vi "WinOption.vi"(8 "error in":errorcluster) -> (0 "error out":errorcluster)   [LabVIEW 2016]
uses:
  Ctl/Option.ctl
panel:
  in  "管理员登录":bool
  in  "选项卡控件":enum32{"基本配置", "流程配置"}(tab)
  in  "Caldata":T1={"分辨率"="", "Fps"=0, "工单号"="", "操作人"="", "增益模式"=enum."高低增益切换", "黑体设定温度1"=0.0, "温差范围1"=0.0, "出图到测温等待时间"=0.0, "调焦数值min"=0, "盲元阈值"=0.0, "盲元采样帧数"=0, "调焦数值min2"=0, "黑体设定温度2"=0.0, "温差范围2"=0.0, "ID选择"=enum."新ID", "快门时间间隔设置"={"快门第一次延时时间"=200, "快门第二次延时时间"=200, "切换增益后快门第一次延时时间"=200, "切换增益后快门第二次延时时间"=200}, "产品名"="Tiny1_C", "镜头"="02011X", "测温功能"="WR", "产品料号"="", "打印机VISA"="", "焦距选择"=enum."Radio Selection 1", "工位"="0001", "服务器保存地址"=path ""}
  in  "Exit":bool
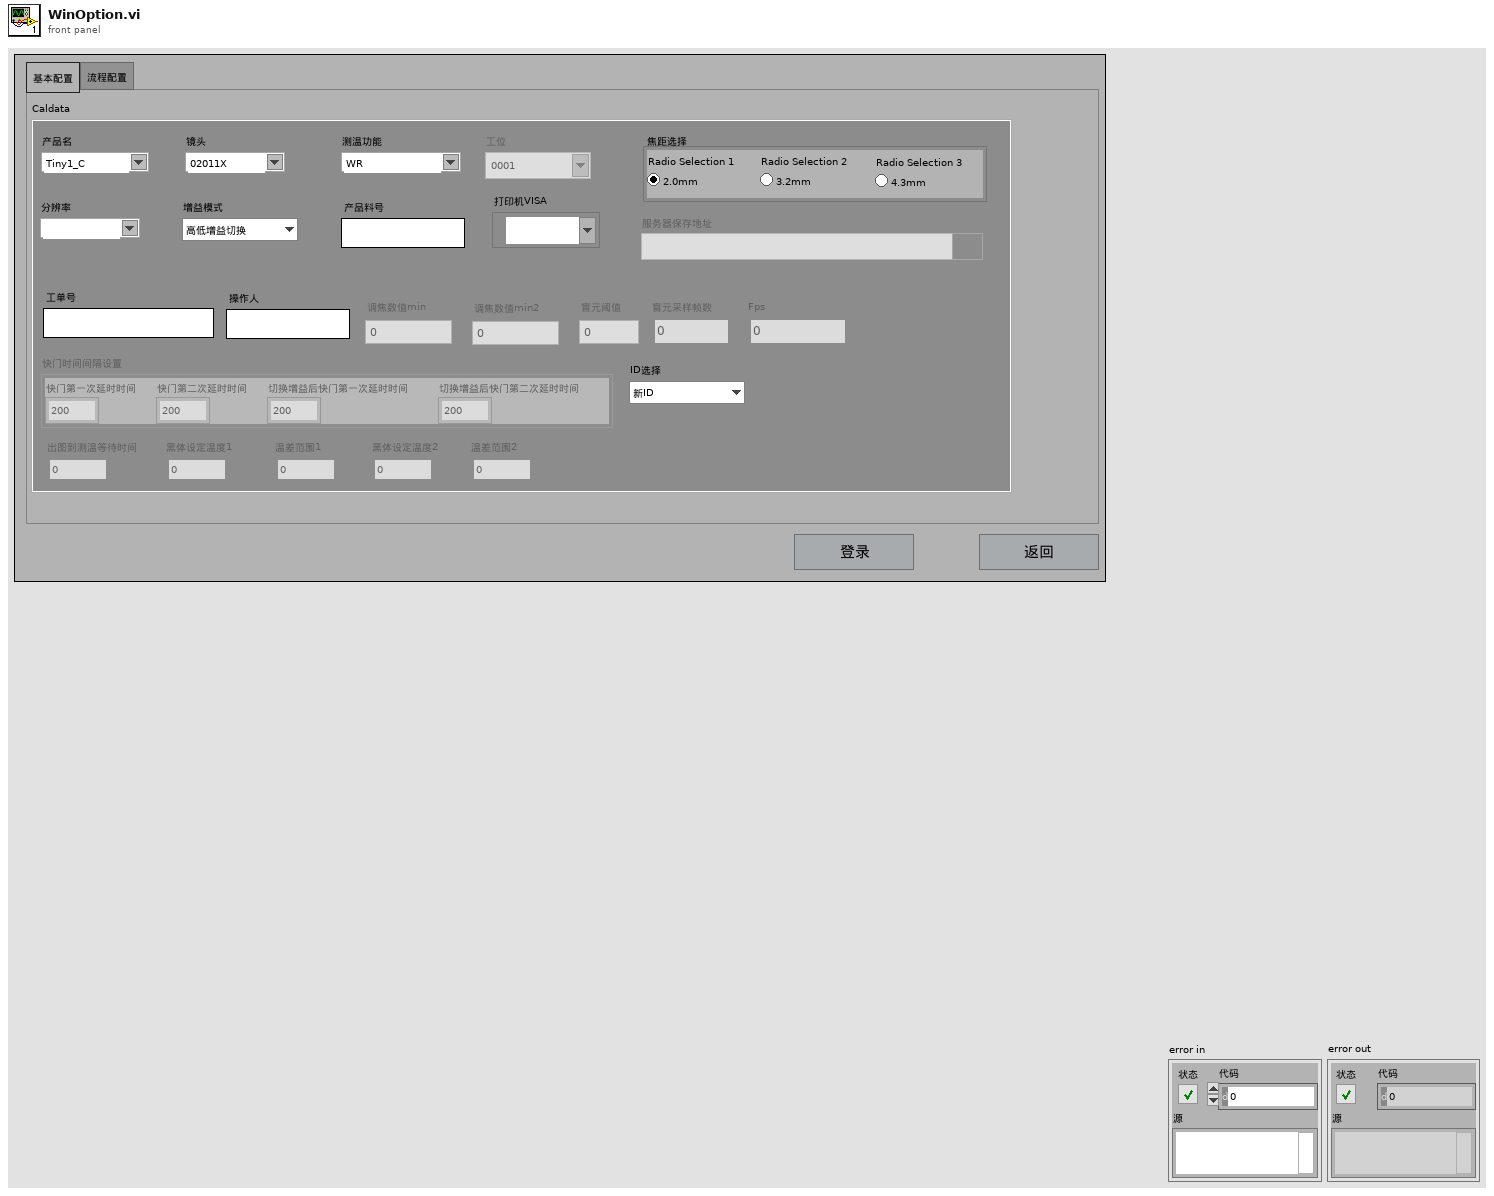
[diagram p1: front panel]
types:
  T1 = typedef "Option.ctl" = cluster{"分辨率":string, "Fps":u16, "工单号":string, "操作人":string, "增益模式":enum16{"高低增益切换", "高增益"}, "黑体设定温度1":dbl, "温差范围1":dbl, "出图到测温等待时间":dbl, "调焦数值min":i32, "盲元阈值":dbl, "盲元采样帧数":u16, "调焦数值min2":i32, "黑体设定温度2":dbl, "温差范围2":dbl, "ID选择":enum16{"旧ID", "新ID"}, "快门时间间隔设置":cluster{"快门第一次延时时间":u16, "快门第二次延时时间":u16, "切换增益后快门第一次延时时间":u16, "切换增益后快门第二次延时时间":u16}, "产品名":string, "镜头":string, "测温功能":string, "产品料号":string, "打印机VISA":refnum<visa-resource-name>, "焦距选择":enum32{"Radio Selection 1", "Radio Selection 2", "Radio Selection 3"}, "工位":string, "服务器保存地址":path}
  T2 = cluster{"CalData":path, "Datasave":path, "Data":path}
  T3 = enum8{"Enabled", "Disabled", "Disabled and Grayed Out"}
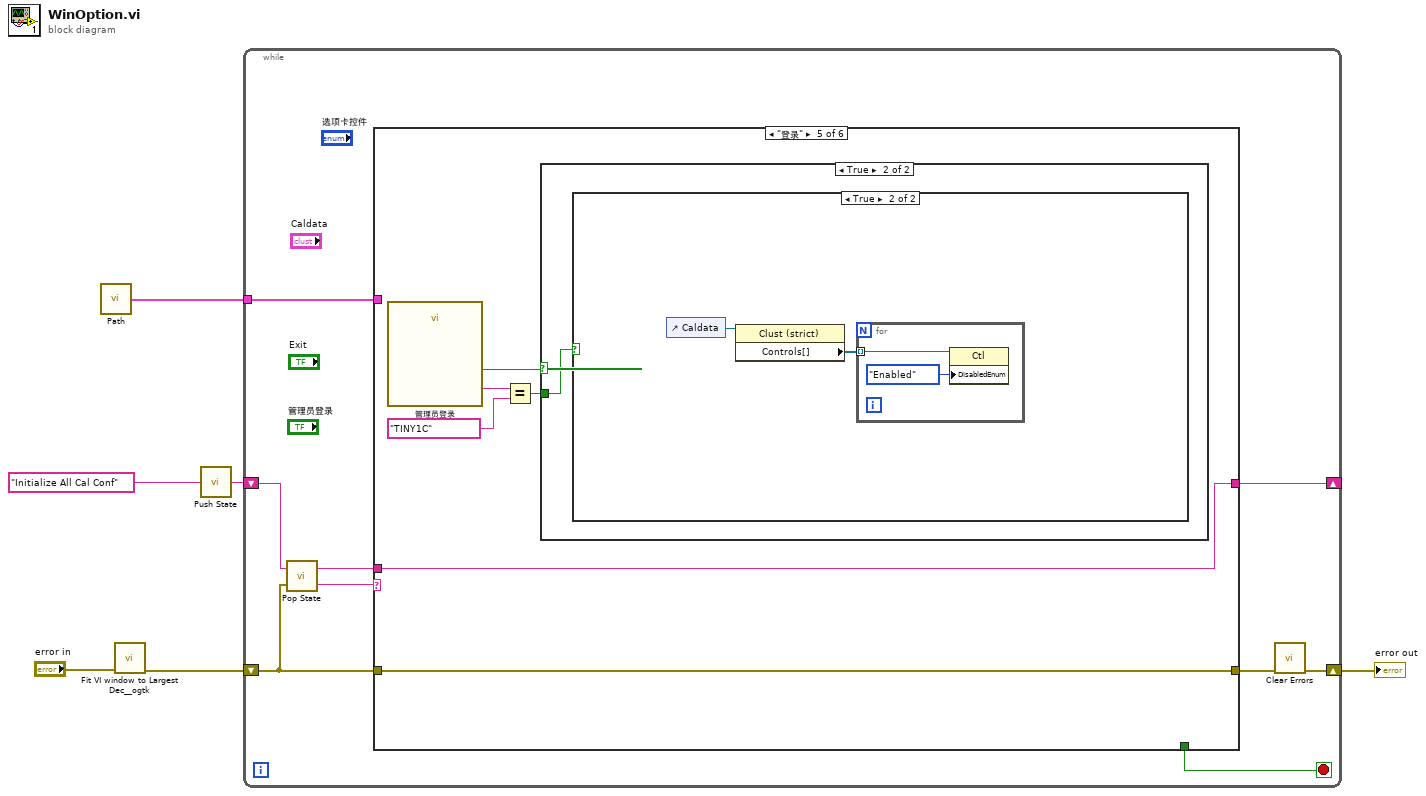
[diagram p0: block diagram]
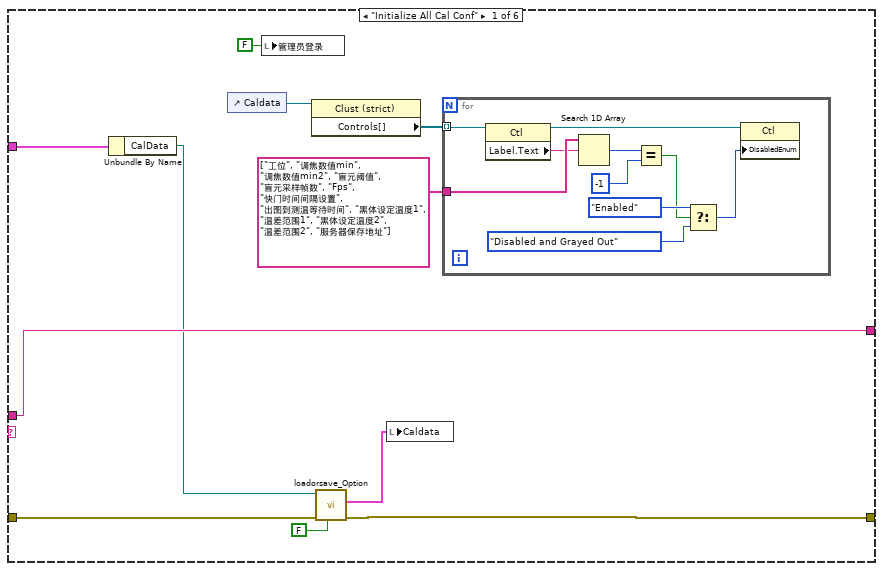
[diagram p2: hidden frame]
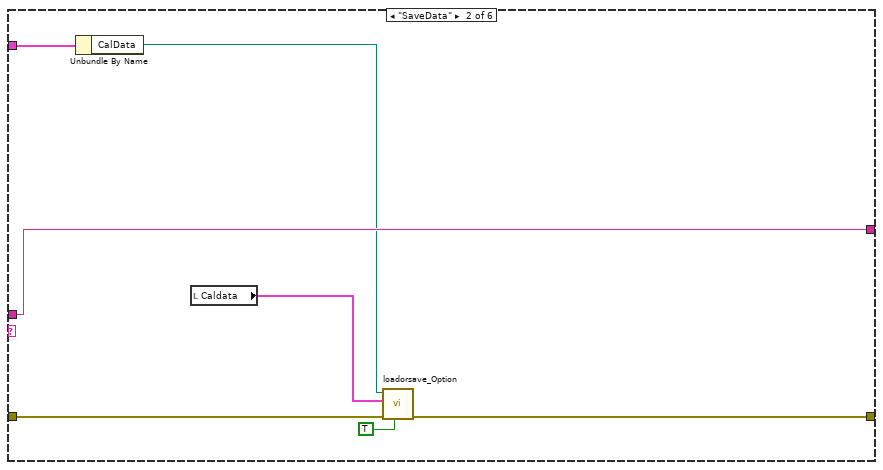
[diagram p3: hidden frame]
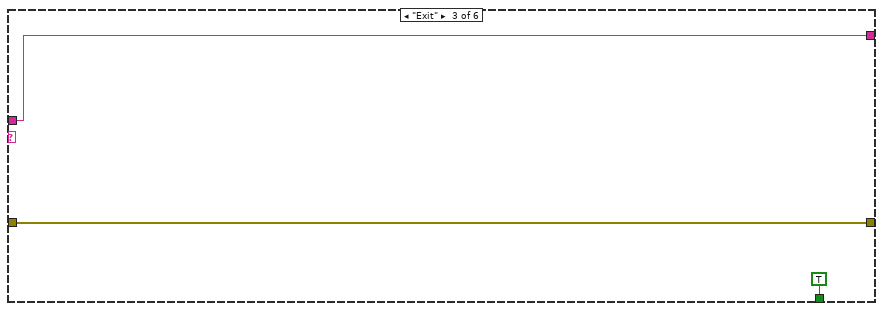
[diagram p4: hidden frame]
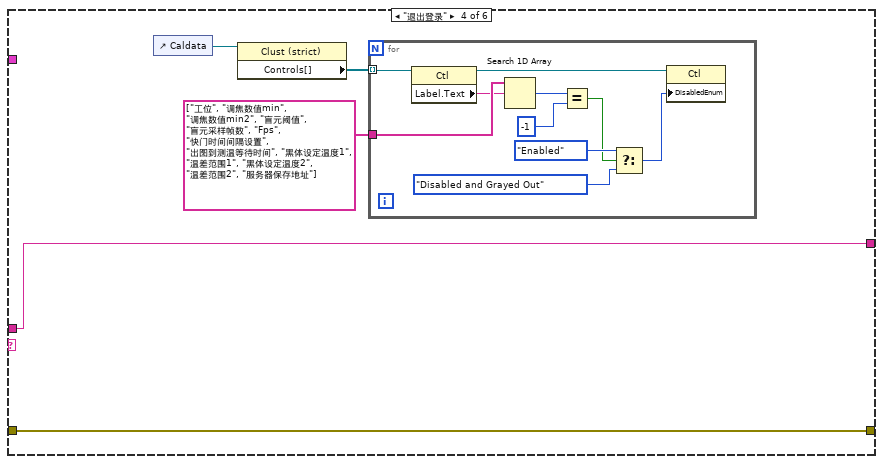
[diagram p5: hidden frame]
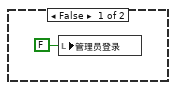
[diagram p6: hidden frame]
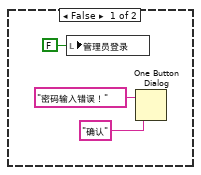
[diagram p7: hidden frame]
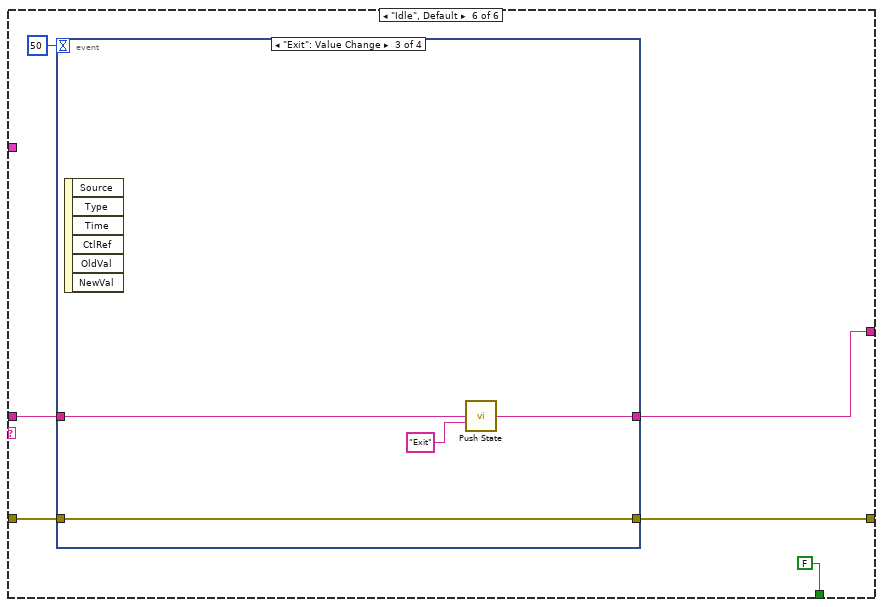
[diagram p8: hidden frame]
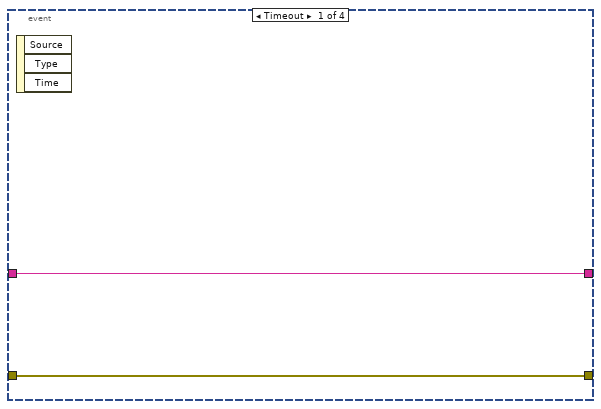
[diagram p9: hidden frame]
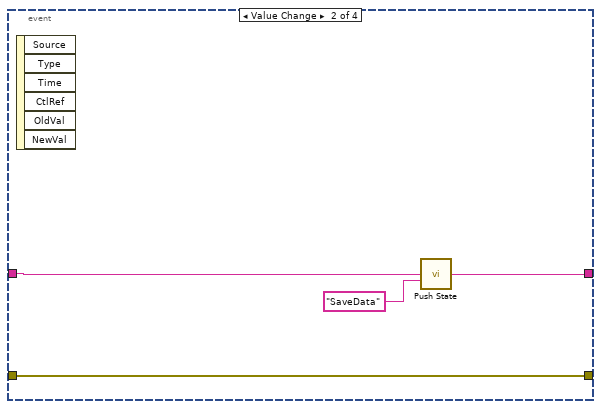
[diagram p10: hidden frame]
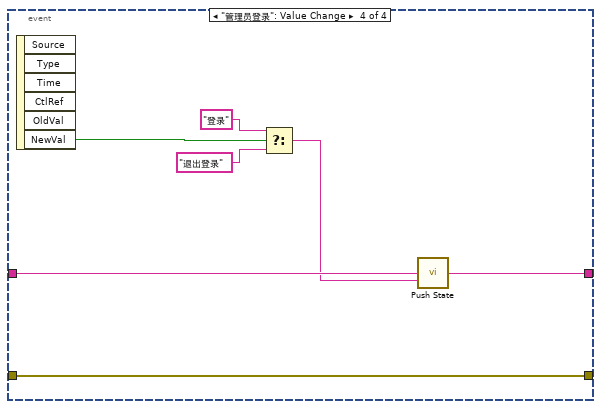
[diagram p11: hidden frame]
diagram:
  n1 = call "Path.vi"() -> ("path"=w1:T2)  [unwired: 9 in]
  n2 = call "Fit VI window to Largest Dec__ogtk.vi"("error in (no error)"="error in") -> ("error out"=w3:errorcluster)  [unwired: 5 in, 1 out]
  n3 = call "Push State.vi"("States In"="Initialize All Cal Conf") -> ("States Out"=w4:string)  [unwired: 14 in]
  n4 = while {
    shift-right: [w11] -> _
    shift-left: w4 -> [w15]
    shift-right: [w9] -> w2
    shift-left: w3 -> [w12]
    tunnel: w1 -> [w8]
    stop <- w7 stop-if-true
    n5 = call "Pop State.vi"("error in (no error)"=w12, "Pre States"=w15) -> ("New State"=w14:string, "Remaining States"=w13:string)
    n6 = case shown="\"登录\"" w14 {
      tunnel: w13 -> [w22 w39 w46 w51 w67 w81]
      tunnel: w12 -> [w26 w43 w45 w50 w66 w80]
      tunnel: [w21 w38 w45 w50 w66 w79] -> w10
      tunnel: [w22 w39 w46 w51 w67 w78] -> w11
      tunnel: w8 -> [w25 w41 _ _ _ _]
      tunnel: [_ _ TRUE _ _ FALSE] -> w7
      frame "Initialize All Cal Conf" {
        n7 = Unbundle By Name(w25) -> ("CalData"=w20:path)
        n8 = control-ref of="Caldata"() -> (w19:refnum<vi>)
        n9 = local write "管理员登录"(FALSE ("管理员登录")) -> ()
        n10 = property class="Clust (strict)"(reference=w19) -> ("Controls[]"=w18:refnum<vi>[])  [unwired: 1 in, 2 out]
        n11 = call "loadorsave_Option.vi"("save?"=FALSE, "error in"=w26, "Path in"=w20) -> ("error out"=w21:errorcluster, "Caldata out"=w24:T1)  [unwired: 6 in, 1 out]
        n12 = local write "Caldata"(w24) -> ()
        n13 = for {
          tunnel: w18 -> [w36] mode=indexing
          tunnel: string[] ["工位", "调焦数值min", "调焦数值min2", "盲元阈值", "盲元采样帧数", "Fps", "快门时间间隔设置", "出图到测温等待时间", "黑体设定温度1", "温差范围1", "黑体设定温度2", "温差范围2", "服务器保存地址"] -> [w35]
          n14 = property class="Ctl"(reference=w36) -> (reference out=w31:refnum<vi>, "Label.Text"=w34:string)  [unwired: 1 in, 1 out]
          n15 = Search 1D Array(1D array=w35, element=w34) -> (index of element=w33:i32)  [unwired: 1 in]
          n16 = Equal?(x=w33, y=-1) -> (x = y?=w28:bool)
          n17 = Select(t=T3."Enabled" ("Disabled"), s=w28, f=T3."Disabled and Grayed Out" ("Disabled")) -> (s? t:f=w27:T3)
          n18 = property class="Ctl"(reference=w31, "DisabledEnum"=w27) -> ()  [unwired: 1 in, 2 out]
        }
      }
      frame "SaveData" {
        n19 = Unbundle By Name(w41) -> ("CalData"=w37:path)
        n20 = local read "Caldata"() -> (w42:T1)
        n21 = call "loadorsave_Option.vi"("save?"=TRUE, "error in"=w43, "Caldata in"=w42, "Path in"=w37) -> ("error out"=w38:errorcluster)  [unwired: 5 in, 2 out]
      }
      frame "Exit" {
      }
      frame "退出登录" {
        n22 = control-ref of="Caldata"() -> (w49:refnum<vi>)
        n23 = property class="Clust (strict)"(reference=w49) -> ("Controls[]"=w48:refnum<vi>[])  [unwired: 1 in, 2 out]
        n24 = for {
          tunnel: w48 -> [w61] mode=indexing
          tunnel: string[] ["工位", "调焦数值min", "调焦数值min2", "盲元阈值", "盲元采样帧数", "Fps", "快门时间间隔设置", "出图到测温等待时间", "黑体设定温度1", "温差范围1", "黑体设定温度2", "温差范围2", "服务器保存地址"] -> [w60]
          n25 = property class="Ctl"(reference=w61) -> (reference out=w56:refnum<vi>, "Label.Text"=w59:string)  [unwired: 1 in, 1 out]
          n26 = Search 1D Array(1D array=w60, element=w59) -> (index of element=w58:i32)  [unwired: 1 in]
          n27 = Equal?(x=w58, y=-1) -> (x = y?=w53:bool)
          n28 = Select(t=T3."Enabled" ("Disabled"), s=w53, f=T3."Disabled and Grayed Out" ("Disabled")) -> (s? t:f=w52:T3)
          n29 = property class="Ctl"(reference=w56, "DisabledEnum"=w52) -> ()  [unwired: 1 in, 2 out]
        }
      }
      frame "登录" {
        n30 = call "管理员登录"() -> ("密码："=w65:string, "确认"=w63:bool)  [unwired: 17 in, 1 out]
        n31 = Equal?(x=w65, y="TINY1C") -> (x = y?=w62:bool)
        n32 = case shown="True" w63 {
          tunnel: w62 -> [_ w69]
          frame False {
            n33 = local write "管理员登录"(FALSE ("管理员登录")) -> ()
          }
          frame True {
            n34 = case shown="True" w69 {
              frame False {
                n35 = local write "管理员登录"(FALSE ("管理员登录")) -> ()
                n36 = One Button Dialog(message="密码输入错误！", button name ("OK")="确认") -> ()  [unwired: 1 out]
              }
              frame True {
                n37 = control-ref of="Caldata"() -> (w74:refnum<vi>)
                n38 = property class="Clust (strict)"(reference=w74) -> ("Controls[]"=w73:refnum<vi>[])  [unwired: 1 in, 2 out]
                n39 = for {
                  tunnel: w73 -> [w76] mode=indexing
                  n40 = property class="Ctl"(reference=w76, "DisabledEnum"=T3."Enabled" ("Disabled")) -> ()  [unwired: 1 in, 2 out]
                }
              }
            }
          }
        }
      }
      frame "Idle", Default {
        n41 = event shown="[2] \"Exit\": Value Change" {
          selector: _ -> [_ _ _ _]
          dyn-events: _ -> [_ _ _ _]
          timeout: 50 -> [_ _ _ _]
          tunnel: w81 -> [w84 w88 w92 w99]
          tunnel: [w84 w86 w90 w98] -> w78
          tunnel: w80 -> [w83 w85 w89 w97]
          tunnel: [w83 w85 w89 w97] -> w79
          event Timeout {
            n42 = event-data() -> ()  [unwired: 1 in, 3 out]
          }
          event Value Change {
            n43 = event-data() -> ()  [unwired: 1 in, 6 out]
            n44 = call "Push State.vi"("States In"=w88, "States End"="SaveData") -> ("States Out"=w86:string)  [unwired: 13 in]
          }
          event "Exit": Value Change {
            n45 = event-data() -> ()  [unwired: 1 in, 6 out]
            n46 = call "Push State.vi"("States In"=w92, "States End"="Exit") -> ("States Out"=w90:string)  [unwired: 13 in]
          }
          event "管理员登录": Value Change {
            n47 = event-data() -> ("NewVal"=w96:bool)  [unwired: 1 in, 5 out]
            n48 = Select(t="登录" ("States End"), s=w96, f="退出登录" ("States End")) -> (s? t:f=w93:string)
            n49 = call "Push State.vi"("States In"=w99, "States End"=w93) -> ("States Out"=w98:string)  [unwired: 13 in]
          }
        }
      }
    }
    n50 = call <vilib>:"Clear Errors.vi"("error in (no error)"=w10) -> ("error out"=w9:errorcluster)  [unwired: 5 in, 1 out]
  }
  "error out" <- w2
